vi "Error_Control.vi"(0 "ERD Loop":refnum<queue>, 1 "GEA2":refnum<queue>, 2 "Command (Handle Errors)":T3=enum."Handle Errors", 5 "Receive Loop":T2, 7 "UI Loop Error":T1, 9 "DAQ":refnum<queue>, 11 "Error In":errorcluster, 12 "Cont Send":refnum<queue>) -> (15 "Error Out":errorcluster)   [LabVIEW 2021]
uses:
  type defs/Error_Command.ctl
  type defs/ERD_Data_Loop_Control.ctl
  type defs/ERD_Loop_States.ctl
  Common/GExplorer Support/typedefs/GExplorer_Data_Cluster.ctl
  type defs/DAQ_States.ctl
  type defs/Ref_ReceiveLoop_Error_UserEvent.ctl
  type defs/Ref_UILoop_Error_UserEvent.ctl
  type defs/Cont_Send_States.ctl
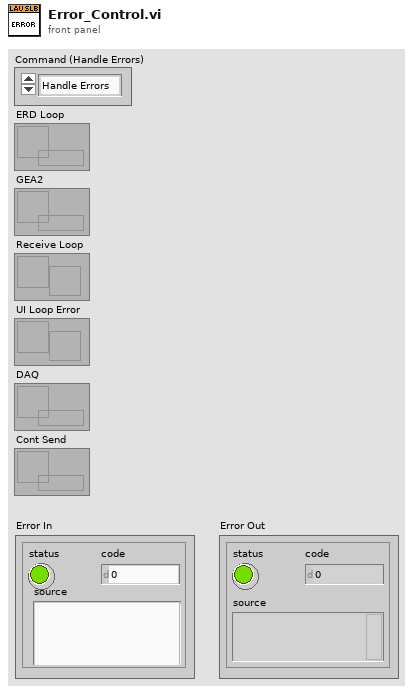
[diagram p1: front panel]
types:
  T1 = typedef "Ref_UILoop_Error_UserEvent.ctl" = refnum<user-event>
  T2 = typedef "Ref_ReceiveLoop_Error_UserEvent.ctl" = refnum<user-event>
  T3 = typedef "Error_Command.ctl" = enum16{"Initialize", "Handle Errors", "Report Errors"}
  T4 = typedef "Cont_Send_States.ctl" = enum16{"Run", "Shutdown"}
  T5 = typedef "DAQ_States.ctl" = enum16{"Wait for Init", "Rename Devices", "Verify Hardware", "Initialize", "Run", "Shutdown", "Exit"}
  T6 = typedef "ERD_Data_Loop_Control.ctl" = cluster{"Data":variant, "State":T7}
  T7 = typedef "ERD_Loop_States.ctl" = enum16{"Init", "Get Version", "Build ERD Read List", "Read ERDs", "Update UI", "Update Graphs", "Read Faults", "Log Data", "Pause", "Brass Logging", "Shutdown"}
  T8 = typedef "GExplorer_Data_Cluster.ctl" = cluster{"Data":variant, "State":enum16{"Add to Log", "Clear", "Shutdown"}}
  T9 = typedef "Ref_ReceiveLoop_UserEvent.ctl" = refnum<user-event>
  T10 = typedef "Ref_UILoop_UserEvent.ctl" = refnum<user-event>
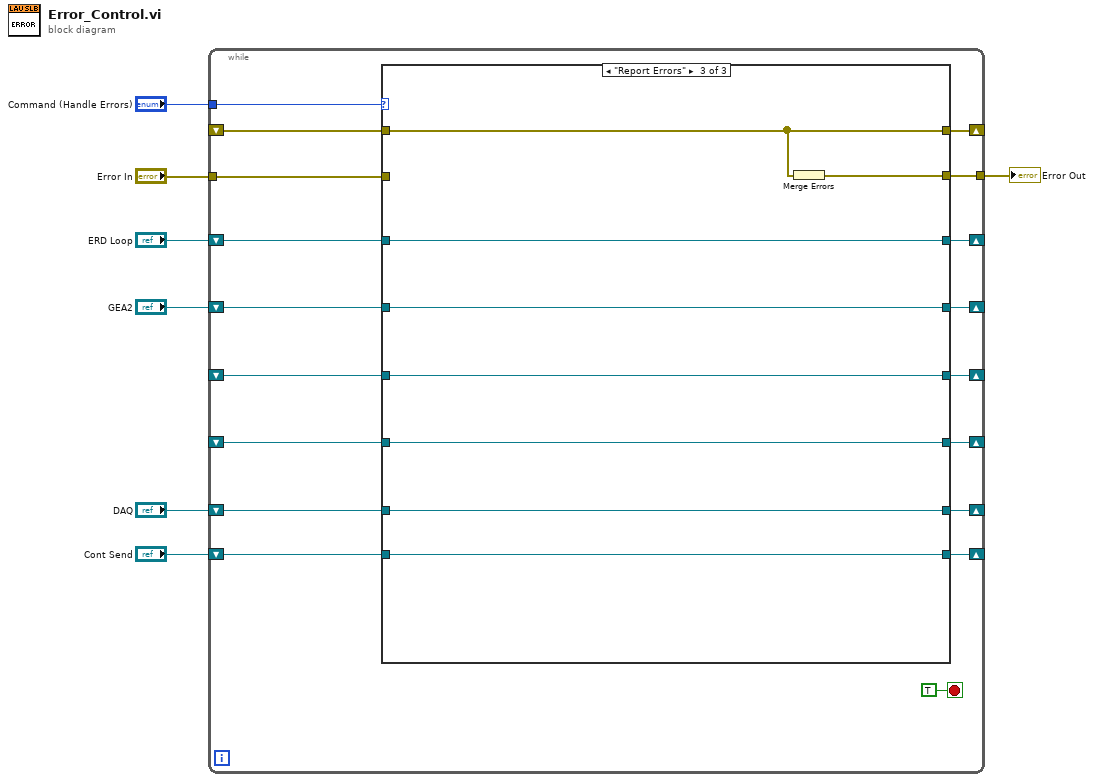
[diagram p0: block diagram]
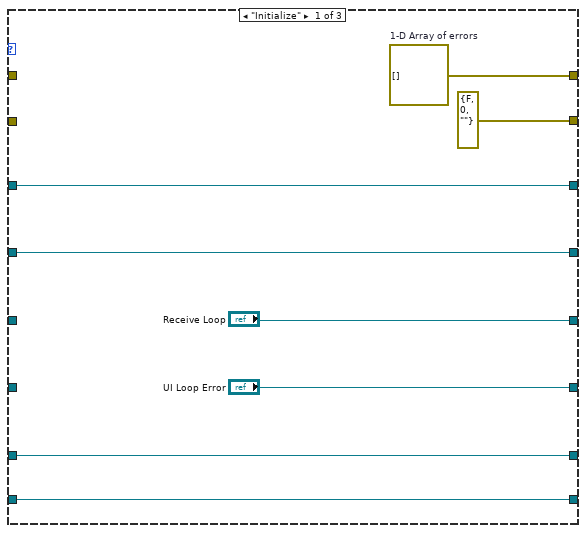
[diagram p2: hidden frame]
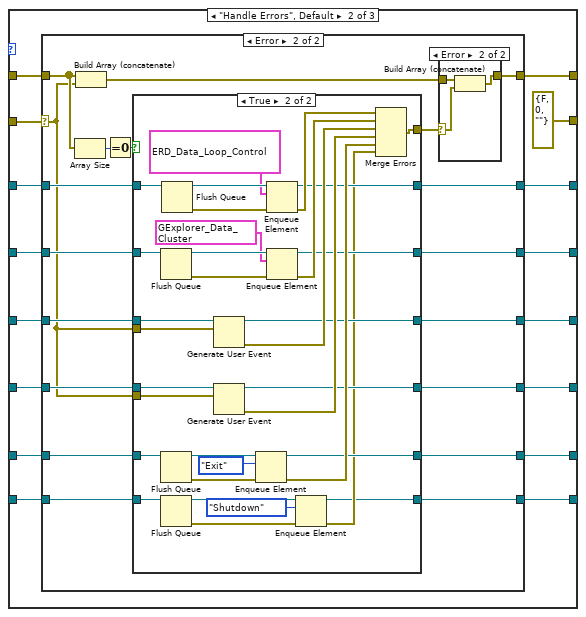
[diagram p3: hidden frame]
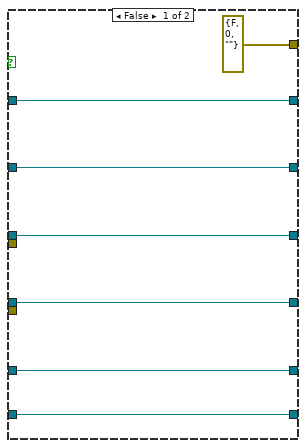
[diagram p5: hidden frame]
diagram:
  n1 = while {
    tunnel: "Error In" -> [w23]
    tunnel: "Command (Handle Errors)" -> [w24]
    shift-right: [w22] -> _
    shift-left: _ -> [w21]
    tunnel: [w20] -> w5
    shift-right: [w19] -> _
    shift-left: "ERD Loop" -> [w14]
    shift-right: [w18] -> _
    shift-left: "GEA2" -> [w13]
    shift-right: [w17] -> _
    shift-left: _ -> [w12]
    shift-right: [w16] -> _
    shift-left: _ -> [w11]
    shift-right: [w15] -> _
    shift-left: "DAQ" -> [w10]
    shift-right: [w9] -> _
    shift-left: "Cont Send" -> [w8]
    stop <- TRUE stop-if-true
    n2 = case shown="\"Report Errors\"" w24 {
      tunnel: w23 -> [_ w49 _]
      tunnel: [w33 w42 w126] -> w22
      tunnel: w21 -> [_ w48 w126]
      tunnel: [errorcluster {"status"=FALSE, "code"=0, "source"=""} ("Error In") errorcluster {"status"=FALSE, "code"=0, "source"=""} ("Error In") w127] -> w20
      tunnel: [w31 w40 w125] -> w19
      tunnel: [w30 w41 w124] -> w18
      tunnel: ["Receive Loop" w39 w123] -> w17
      tunnel: ["UI Loop Error" w38 w122] -> w16
      tunnel: [w29 w37 w121] -> w15
      tunnel: w14 -> [w31 w47 w125]
      tunnel: w13 -> [w30 w46 w124]
      tunnel: w12 -> [_ w45 w123]
      tunnel: w11 -> [_ w44 w122]
      tunnel: w10 -> [w29 w43 w121]
      tunnel: [w26 w34 w120] -> w9
      tunnel: w8 -> [w26 w35 w120]
      frame "Initialize" {
        w33 = errorcluster[] []  # 1-D Array of errors
      }
      frame "Handle Errors", Default {
        n3 = case shown="Error" w49 {
          selector: w49 -> [_ w65]
          tunnel: w48 -> [w56 w75]
          tunnel: w47 -> [w55 w72]
          tunnel: w46 -> [w54 w71]
          tunnel: w45 -> [w53 w70]
          tunnel: w44 -> [w52 w69]
          tunnel: w43 -> [w51 w68]
          tunnel: [w56 w66] -> w42
          tunnel: [w54 w64] -> w41
          tunnel: [w55 w63] -> w40
          tunnel: [w53 w62] -> w39
          tunnel: [w52 w61] -> w38
          tunnel: [w51 w60] -> w37
          tunnel: w35 -> [w50 w58]
          tunnel: [w50 w57] -> w34
          frame No Error {
          }
          frame Error {
            n4 = Array Size(array=w75) -> (size(s)=w74:i32)
            n5 = Build Array (concatenate)(w75, w65) -> (w59:errorcluster[])
            n6 = Equal To 0?(x=w74) -> (x = 0?=w73:bool)
            n7 = case shown="True" w73 {
              tunnel: w72 -> [w81 w115]
              tunnel: w71 -> [w80 w114]
              tunnel: w70 -> [w79 w105]
              tunnel: w69 -> [w78 w103]
              tunnel: w68 -> [w77 w113]
              tunnel: [errorcluster {"status"=FALSE, "code"=0, "source"=""} ("error IO") w112] -> w67
              tunnel: w65 -> [_ w104]
              tunnel: w65 -> [_ w102]
              tunnel: [w80 w94] -> w64
              tunnel: [w81 w93] -> w63
              tunnel: [w79 w92] -> w62
              tunnel: [w78 w91] -> w61
              tunnel: [w77 w90] -> w60
              tunnel: w58 -> [w76 w88]
              tunnel: [w76 w83] -> w57
              frame False {
              }
              frame True {
                n8 = Flush Queue(queue=w114) -> (queue out=w110:refnum<queue>, error out=w111:errorcluster)  [unwired: 1 in, 1 out]
                n9 = Flush Queue(queue=w113) -> (queue out=w101:refnum<queue>, error out=w100:errorcluster)  [unwired: 1 in, 1 out]
                n10 = Flush Queue(queue=w88) -> (queue out=w86:refnum<queue>, error out=w87:errorcluster)  [unwired: 1 in, 1 out]
                n11 = Flush Queue(queue=w115) -> (queue out=w107:refnum<queue>, error out=w108:errorcluster)  [unwired: 1 in, 1 out]
                n12 = Generate User Event(user event=w105, event data cluster=w104) -> (user event out=w92:T9, error out=w97:errorcluster)  [unwired: 2 in]
                n13 = Generate User Event(user event=w103, event data cluster=w102) -> (user event out=w91:T10, error out=w98:errorcluster)  [unwired: 2 in]
                n14 = Enqueue Element(queue=w101, element=DAQ_States."Exit", error in (no error)=w100) -> (queue out=w90:refnum<queue>, error out=w99:errorcluster)  [unwired: 1 in, 1 out]
                n15 = Enqueue Element(queue=w107, element=T6 {"Data"=variant, "State"=enum."Shutdown"}, error in (no error)=w108) -> (queue out=w93:refnum<queue>, error out=w96:errorcluster)  [unwired: 1 in, 1 out]
                n16 = Enqueue Element(queue=w110, element=T8 {"Data"=variant, "State"=enum."Shutdown"}, error in (no error)=w111) -> (queue out=w94:refnum<queue>, error out=w95:errorcluster)  [unwired: 1 in, 1 out]
                n17 = Enqueue Element(queue=w86, element=Cont_Send_States."Shutdown", error in (no error)=w87) -> (queue out=w83:refnum<queue>, error out=w84:errorcluster)  [unwired: 1 in, 1 out]
                n18 = Merge Errors(w96, w95, w97, w98, w99, w84) -> (w112:errorcluster)
              }
            }
            n19 = case shown="Error" w67 {
              selector: w67 -> [_ w118]
              tunnel: [w116 w119] -> w66
              tunnel: w59 -> [w116 w117]
              frame No Error {
              }
              frame Error {
                n20 = Build Array (concatenate)(w117, w118) -> (w119:errorcluster[])
              }
            }
          }
        }
      }
      frame "Report Errors" {
        n21 = Merge Errors(w126) -> (w127:errorcluster)
      }
    }
  }
  "Error Out" <- w5
